vi "Test Clusters and Init.vi"() -> ()   [LabVIEW 2013]
uses:
  My circular buffer info.ctl
panel:
  in  "stop":bool
  out "read buffer ref queue":refnum<queue>
  out "Event delay queue":refnum<queue>
  out "command queue":refnum<queue>
  out "samples/block/channel 2":i32
  out "number of channels 2":i32
  out "bytes/sample 2":i32
  out "blocks/event":i32
  out "samples/block":i32
  out "num blocks after 2":i32
  out "num blocks  prior 2":i32
  out "xml header":string
  out "archive directory 2":path
  out "buffer2 path 2":path
  out "buffer1 path 2":path
  out "buff ref2":refnum<file>
  out "buff ref1":refnum<file>
  in  "buffer2 path":path
  in  "buffer1 path":path
  in  "archive directory":path
  in  "num blocks  prior":i32
  in  "num blocks after":i32
  in  "bytes/sample":i32
  in  "samples/block/channel":i32
  in  "number of channels":i32
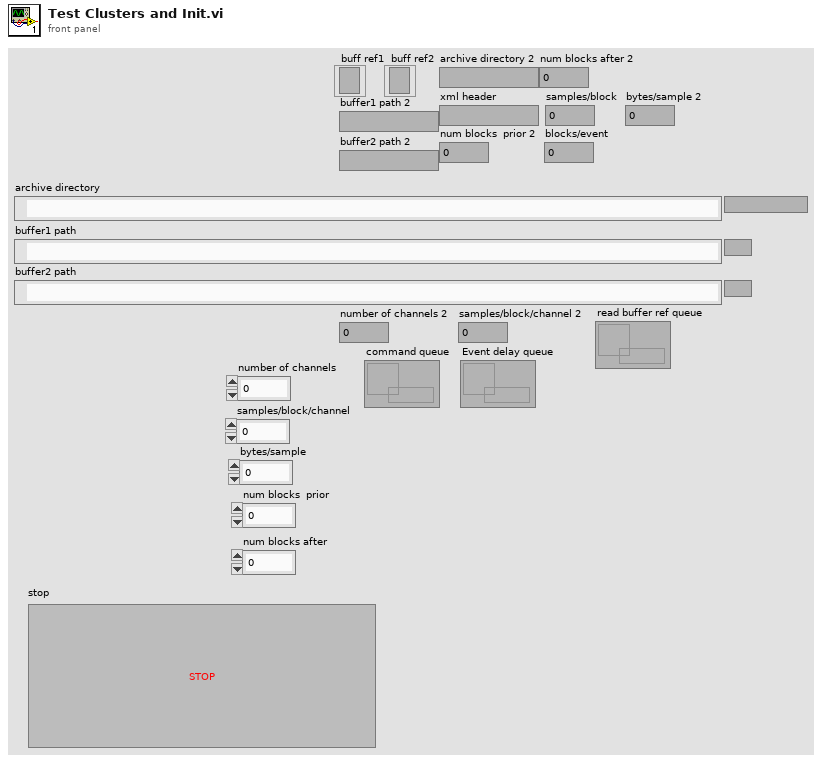
[diagram p1: front panel]
types:
  T1 = typedef "My circular buffer info.ctl" = cluster{"buff ref1":refnum<file>, "buff ref2":refnum<file>, "buffer1 path":path, "buffer2 path":path, "archive directory":path, "xml header":string, "num blocks  prior":i32, "num blocks after":i32, "blocks/event":i32, "samples/block":i32, "bytes/sample":i32, "number of channels":i32, "samples/block/channel":i32, "read buffer ref queue":refnum<queue>, "Event delay queue":refnum<queue>, "command queue":refnum<queue>}
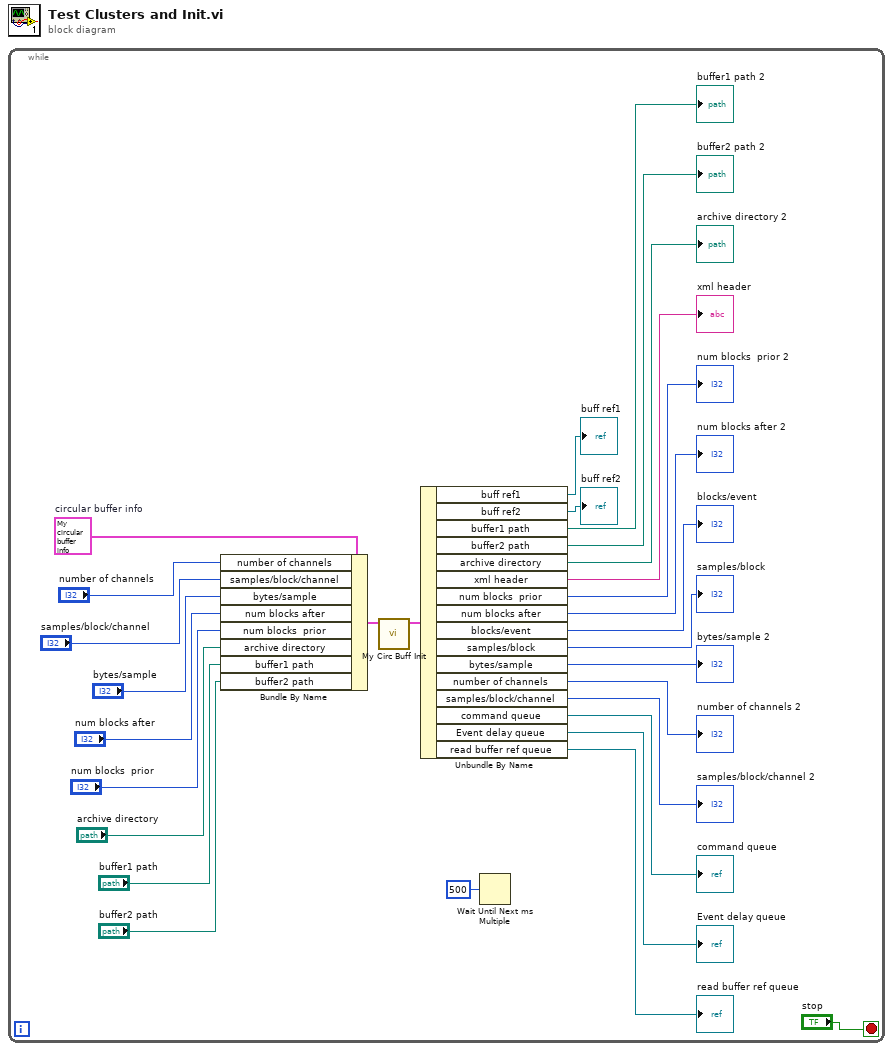
[diagram p0: block diagram]
diagram:
  n1 = while {
    stop <- "stop" stop-if-true
    w24 = T1 {"buff ref1"=refnum, "buff ref2"=refnum, "buffer1 path"=path "", "buffer2 path"=path "", "archive directory"=path "", "xml header"="", "num blocks  prior"=0, "num blocks after"=0, "blocks/event"=0, "samples/block"=0, "bytes/sample"=0, "number of channels"=0, "samples/block/channel"=0, "read buffer ref queue"=refnum, "Event delay queue"=refnum, "command queue"=refnum}  # circular buffer info
    n2 = Bundle By Name(cluster=w24, "number of channels"="number of channels", "samples/block/channel"="samples/block/channel", "bytes/sample"="bytes/sample", "num blocks after"="num blocks after", "num blocks  prior"="num blocks  prior", "archive directory"="archive directory", "buffer1 path"="buffer1 path", "buffer2 path"="buffer2 path") -> (w20:T1)
    n3 = call "My Circ Buff Init.vi"("circular buffer info"=w20) -> ("circular buffer info out"=w19:T1)  [unwired: 9 in, 1 out]
    n4 = Unbundle By Name(w19) -> ("buff ref1"=→"buff ref1":refnum<file>, "buff ref2"=→"buff ref2":refnum<file>, "buffer1 path"=→"buffer1 path 2":path, "buffer2 path"=→"buffer2 path 2":path, "archive directory"=→"archive directory 2":path, "xml header"=→"xml header":string, "num blocks  prior"=→"num blocks  prior 2":i32, "num blocks after"=→"num blocks after 2":i32, "blocks/event"=→"blocks/event":i32, "samples/block"=→"samples/block":i32, "bytes/sample"=→"bytes/sample 2":i32, "number of channels"=→"number of channels 2":i32, "samples/block/channel"=→"samples/block/channel 2":i32, "command queue"=→"command queue":refnum<queue>, "Event delay queue"=→"Event delay queue":refnum<queue>, "read buffer ref queue"=→"read buffer ref queue":refnum<queue>)
    n5 = Wait Until Next ms Multiple(millisecond multiple=u32 500) -> ()  [unwired: 1 out]
  }
